vi "CAN Data Playback.vi"(11 "Source":path=path "C:/Data for Processing/150215 132046.tdms") -> ()   [LabVIEW 2014]
uses:
  <vilib>/RioEmbeddedCAN/RioEmbeddedCAN.llb/CANFrameControl.ctl
  8byte to 4 2byte.vi
  Decode VSM.vi
  Decode Inverter State.vi
  Decode Inverter Enable States.vi
  Decode Inverter Command Modes.vi
  MC/Process Run Fault.vi
  BMS/Decode Car State.vi
  BMS/Scale Cell Voltage.vi
  BMS/Scale Cell Temp.vi
  Global Data.vi
  BMS/Decode Charging State.vi
panel:
  out "error out 2":errorcluster={"status"=TRUE, "code"=118, "source"="TDMS Open in CAN Data Playback.vi"}
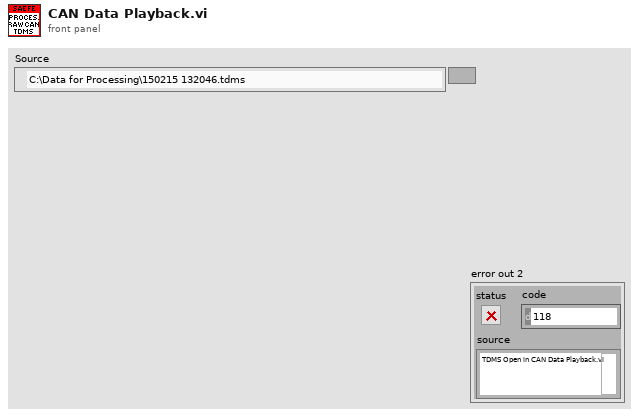
[diagram p1: front panel]
types:
  T1 = typedef "CANFrameControl.ctl" = cluster{"identifier":u32, "extended?":bool, "type":u8, "payload":u8[]}
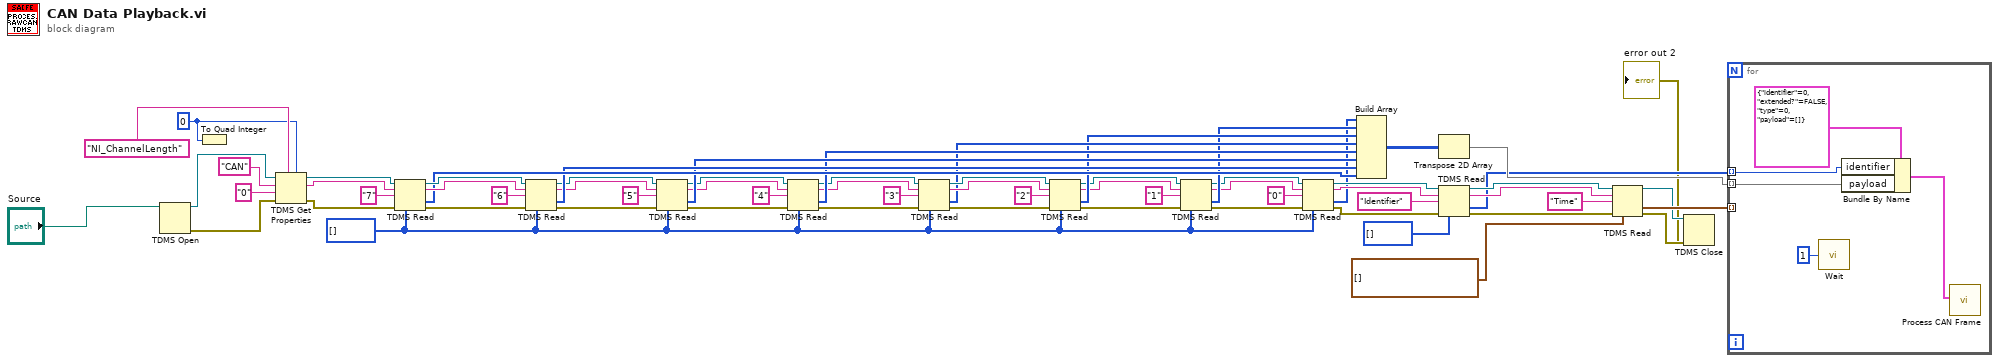
[diagram p0: block diagram]
diagram:
  w9 = u8[] []
  w59 = u64 0 ("data type")
  n1 = TDMS Open(11:"Source") -> (0:w64:errorcluster, 3:w65:refnum<k34>)  [unwired: 6 in]
  n2 = To Quad Integer(1:w59) -> ()  [unwired: 1 out]
  n3 = TDMS Get Properties(5:w59, 7:"NI_ChannelLength" ("property name"), 8:w64, 9:"0" ("channel name"), 10:"CAN" ("group name"), 11:w65) -> (0:w57:errorcluster, 2:w56:string, 3:w58:refnum<k34>)  [unwired: 3 out]
  n4 = TDMS Read(0:w58, 5:w56, 7:"7" ("channel name(s) in"), 11:w57, 12:w9) -> (4:w54:refnum<k34>, 6:w52:string, 10:w50:u8[], 15:w53:errorcluster)  [unwired: 3 in, 2 out]
  n5 = TDMS Read(0:w54, 5:w52, 7:"6" ("channel name(s) in"), 11:w53, 12:w9) -> (4:w48:refnum<k34>, 6:w46:string, 10:w49:u8[], 15:w47:errorcluster)  [unwired: 3 in, 2 out]
  n6 = TDMS Read(0:w48, 5:w46, 7:"5" ("channel name(s) in"), 11:w47, 12:w9) -> (4:w43:refnum<k34>, 6:w42:string, 10:w44:u8[], 15:w40:errorcluster)  [unwired: 3 in, 2 out]
  n7 = TDMS Read(0:w43, 5:w42, 7:"4" ("channel name(s) in"), 11:w40, 12:w9) -> (4:w38:refnum<k34>, 6:w36:string, 10:w39:u8[], 15:w37:errorcluster)  [unwired: 3 in, 2 out]
  n8 = TDMS Read(0:w38, 5:w36, 7:"3" ("channel name(s) in"), 11:w37, 12:w9) -> (4:w34:refnum<k34>, 6:w32:string, 10:w29:u8[], 15:w33:errorcluster)  [unwired: 3 in, 2 out]
  n9 = TDMS Read(0:w34, 5:w32, 7:"2" ("channel name(s) in"), 11:w33, 12:w9) -> (4:w11:refnum<k34>, 6:w5:string, 10:w28:u8[], 15:w10:errorcluster)  [unwired: 3 in, 2 out]
  n10 = TDMS Read(0:w11, 5:w5, 7:"1" ("channel name(s) in"), 11:w10, 12:w9) -> (4:w4:refnum<k34>, 6:w2:string, 10:w8:u8[], 15:w3:errorcluster)  [unwired: 3 in, 2 out]
  n11 = TDMS Read(0:w4, 5:w2, 7:"0" ("channel name(s) in"), 11:w3, 12:w9) -> (4:w27:refnum<k34>, 6:w25:string, 10:w7:u8[], 15:w26:errorcluster)  [unwired: 3 in, 2 out]
  n12 = Build Array(w7, w8, w28, w29, w39, w44, w49, w50) -> (w17:u8[][])
  n13 = Transpose 2D Array(2D array=w17) -> (transposed array=w16:u8[][])
  n14 = TDMS Read(0:w27, 5:w25, 7:"Identifier" ("channel name(s) in"), 11:w26, 12:u32[] []) -> (4:w22:refnum<k34>, 6:w20:string, 10:w14:u32[], 15:w21:errorcluster)  [unwired: 3 in, 2 out]
  n15 = TDMS Read(0:w22, 5:w20, 7:"Time" ("channel name(s) in"), 11:w21, 12:timestamp[] []) -> (4:w13:refnum<k34>, 10:w15:timestamp[], 15:w12:errorcluster)  [unwired: 3 in, 3 out]
  n16 = TDMS Close(8:w12, 11:w13) -> (0:→"error out 2":errorcluster)  [unwired: 1 out]
  n17 = for {
    tunnel: w16 -> [w69] mode=indexing
    tunnel: w15 -> [_] mode=indexing
    tunnel: w14 -> [w68] mode=indexing
    n18 = call "Wait"("Count(mSec)"=u32 1) -> ()  [unwired: 1 out]
    n19 = Bundle By Name(cluster=T1 {"identifier"=0, "extended?"=FALSE, "type"=0, "payload"=[]} ("CAN frame"), "identifier"=w68, "payload"=w69) -> (w67:T1)
    n20 = call "Process CAN Frame.vi"("CAN frame"=w67) -> ()  [unwired: 11 in]
  }
